vi "Shared Variable Main Page.vi"(8 "error in (no error)":errorcluster, 11 "Node Ptr":T1 format="%.0x") -> (0 "error out":errorcluster)   [LabVIEW 2012, in "Shared Variable Custom Device.lvlib"]
uses:
  Shared Variable Custom Device.lvlib
  <vilib>/NI Veristand/Custom Device API/Custom Device Item Ref.ctl
  <vilib>/NI Veristand/Custom Device API/Custom Device API.lvlib
panel:
  in  "Timeout (ms)":i32
  in  "IP Address":string
  in  "Header":cluster{"Section Name":string}={"Section Name"="Custom Device Item Settings"}
  in  "Description":string
  in  "Name":string
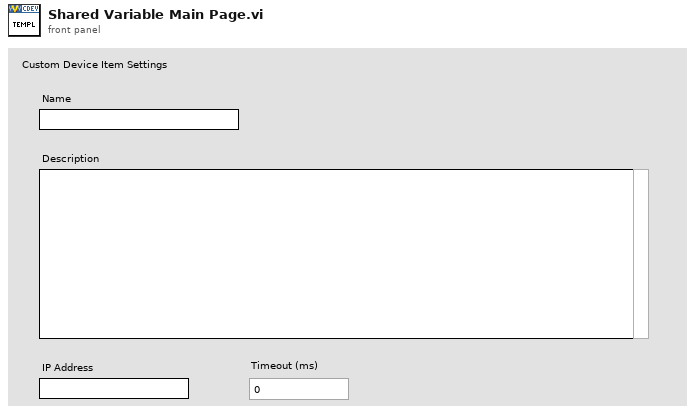
[diagram p1: front panel]
types:
  T1 = typedef "Custom Device API.lvlib/Custom Device Item Ref.ctl" = u64
  T2 = typedef "Custom Device API.lvlib/Custom Device Item Info.ctl" = cluster{"Name":string, "Is Channel":bool, "GUID":string, "Is Waveform":bool}
  T3 = typedef "Custom Device API.lvlib/Custom Device Commands.ctl" = enum16{"Default", "Item renamed", "Shutdown", "Dynamic button pressed"}
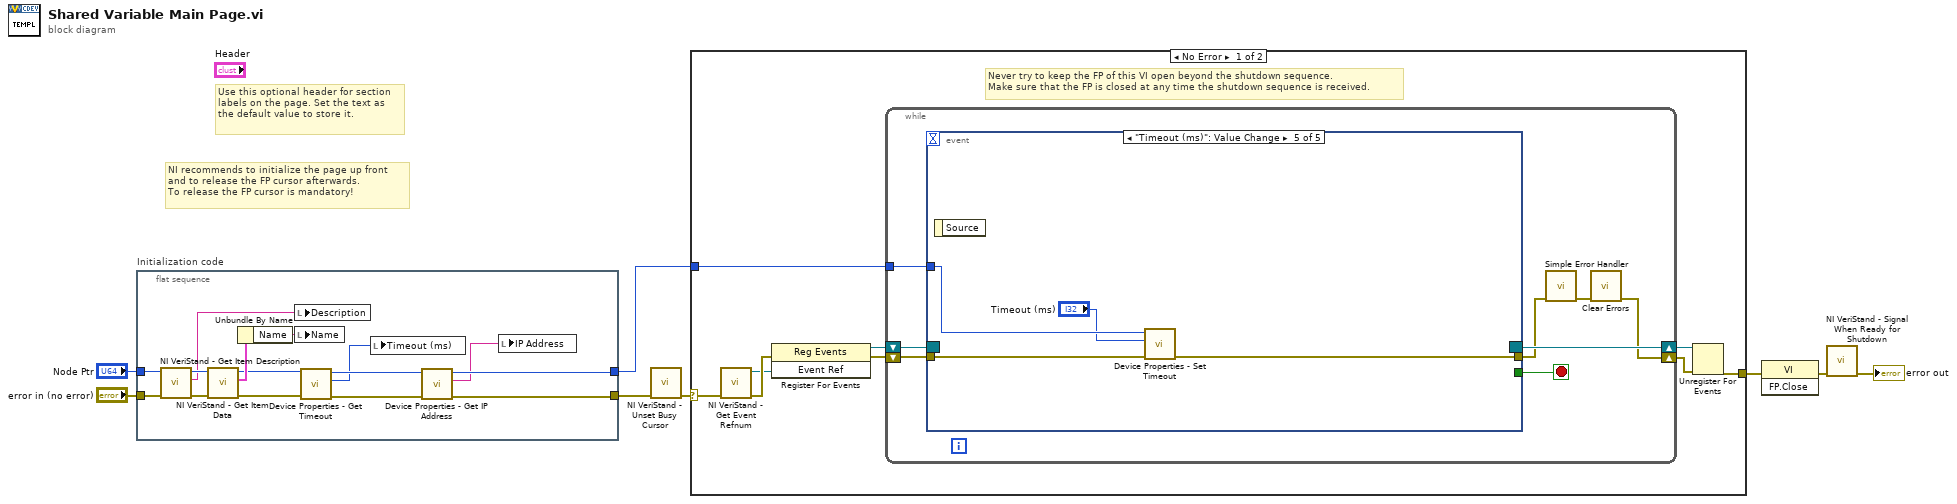
[diagram p0: block diagram]
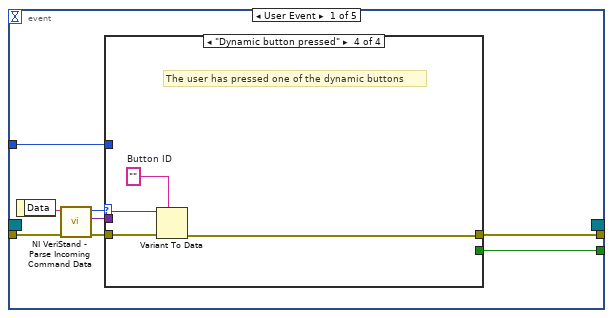
[diagram p2: hidden frame]
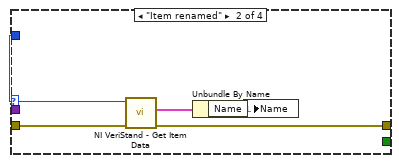
[diagram p4: hidden frame]
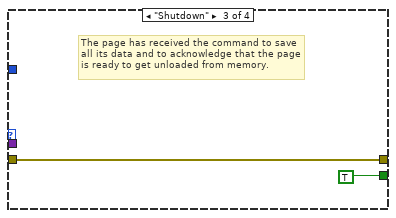
[diagram p5: hidden frame]
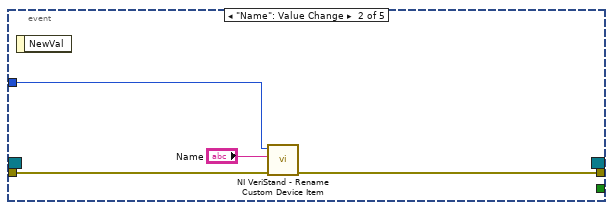
[diagram p6: hidden frame]
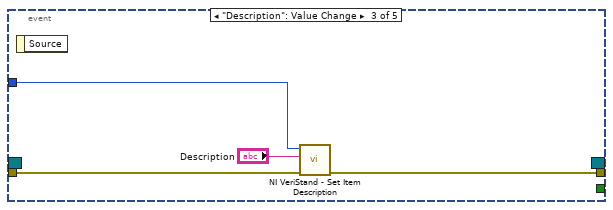
[diagram p7: hidden frame]
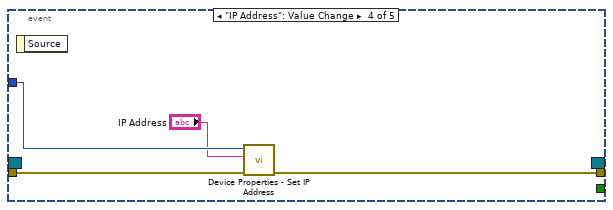
[diagram p8: hidden frame]
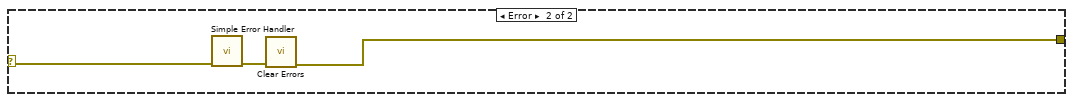
[diagram p9: hidden frame]
diagram:
  # "Use this optional header for section labels on the page. Set the text as the default value to store it."
  # "NI recommends to initialize the page up front\nand to release the FP cursor afterwards.\nTo release the FP cursor is mandatory!"
  n1 = flat-sequence "Initialization code" {
    tunnel: "error in (no error)" -> [w22]
    tunnel: "Node Ptr" -> [w21]
    tunnel: [w10] -> w4
    tunnel: [w11] -> w1
    frame #0 {
      n2 = call <vilib>:"NI VeriStand - Get Item Description.vi"("error in (no error)"=w22, "Item Ref in"=w21) -> ("error out"=w19:errorcluster, "Description"=w20:string, "Item Ref out"=w23:T1)  [unwired: 7 out]
      n3 = call <vilib>:"NI VeriStand - Get Item Data.vi"("error in (no error)"=w19, "Item Ref in"=w23) -> ("error out"=w15:errorcluster, "Item Info"=w18:T2, "Item Ref out"=w16:T1)  [unwired: 7 out]
      n4 = Unbundle By Name(w18) -> ("Name"=w17:string)
      n5 = local write "Description"(w20) -> ()
      n6 = local write "Name"(w17) -> ()
      n7 = call "Device Properties - Get Timeout.vi"("error in (no error)"=w15, "Device Ref in"=w16) -> ("error out"=w14:errorcluster, "IP Address"=w12:i32, "Device Ref out"=w13:T1)  [unwired: 7 in]
      n8 = local write "Timeout (ms)"(w12) -> ()
      n9 = call "Device Properties - Get IP Address.vi"("error in (no error)"=w14, "Device Ref in"=w13) -> ("error out"=w10:errorcluster, "IP Address"=w9:string, "Device Ref out"=w11:T1)  [unwired: 7 in]
      n10 = local write "IP Address"(w9) -> ()
    }
  }
  n11 = call <vilib>:"NI VeriStand - Unset Busy Cursor.vi"("error in (no error)"=w4) -> ("error out"=w3:errorcluster)  [unwired: 10 out]
  n12 = case shown="No Error" w3 {
    selector: w3 -> [w24 w79]
    tunnel: [w29 w77] -> w8
    tunnel: w1 -> [w25 _]
    frame No Error {
      # "Never try to keep the FP of this VI open beyond the shutdown sequence.\nMake sure that the FP is closed at any time the shutdown sequence is received."
      n13 = call <vilib>:"NI VeriStand - Get Event Refnum.vi"("error in (no error)"=w24) -> ("error out"=w32:errorcluster, "Event Ref"=w28:refnum<user-event>)  [unwired: 9 out]
      n14 = register-events(error in=w32, w28) -> (reference out=w26:refnum<event-registration>, error out=w27:errorcluster)  [unwired: 1 in]
      n15 = while {
        tunnel: w25 -> [w36]
        shift-right: [w33] -> w30
        shift-left: w27 -> [w39]
        shift-right: [w40] -> w31
        shift-left: w26 -> [w38]
        stop <- w37 stop-if-true
        n16 = event shown="[4] \"Timeout (ms)\": Value Change" {
          selector: w38 -> [_ _ _ _ _]
          dyn-events: [_ _ _ _ _] -> w40
          timeout: _ -> [_ _ _ _ _]
          tunnel: w39 -> [w48 w64 w67 w72 w76]
          tunnel: [w44 _ _ _ _] -> w37
          tunnel: [w43 w63 w66 w69 w73] -> w35
          tunnel: w36 -> [w42 w62 w68 w71 w75]
          event User Event {
            n17 = event-data() -> ("Data"=w47:string)  [unwired: 1 out]
            n18 = call <vilib>:"NI VeriStand - Parse Incoming Command Data.vi"("error in (no error)"=w48, "Incoming data"=w47) -> ("error out"=w46:errorcluster, "Outgoing data"=w41:variant, "Action"=w45:T3)  [unwired: 7 out]
            n19 = case shown="\"Dynamic button pressed\"" w45 {
              tunnel: w46 -> [w49 w54 w55 w60]
              tunnel: [_ _ TRUE _] -> w44
              tunnel: [w49 w51 w55 w57] -> w43
              tunnel: w42 -> [_ w53 _ _]
              tunnel: w41 -> [_ _ _ w59]
              frame "Default", Default {
              }
              frame "Item renamed" {
                n20 = call <vilib>:"NI VeriStand - Get Item Data.vi"("error in (no error)"=w54, "Item Ref in"=w53) -> ("error out"=w51:errorcluster, "Item Info"=w52:T2)  [unwired: 8 out]
                n21 = Unbundle By Name(w52) -> ("Name"=w50:string)
                n22 = local write "Name"(w50) -> ()
              }
              frame "Shutdown" {
                # "The page has received the command to save all its data and to acknowledge that the page is ready to get unloaded from memory."
              }
              frame "Dynamic button pressed" {
                w58 = ""  # Button ID
                # "The user has pressed one of the dynamic buttons"
                n23 = Variant To Data(error in=w60, type=w58, Variant=w59) -> (error out=w57:errorcluster)  [unwired: 1 out]
              }
            }
          }
          event "Name": Value Change {
            n24 = event-data() -> ()  [unwired: 2 out]
            n25 = call <vilib>:"NI VeriStand - Rename Custom Device Item.vi"("error in (no error)"=w64, "New Name"="Name", "Item Ref in"=w62) -> ("error out"=w63:errorcluster)  [unwired: 1 in, 7 out]
          }
          event "Description": Value Change {
            n26 = event-data() -> ()  [unwired: 2 out]
            n27 = call <vilib>:"NI VeriStand - Set Item Description.vi"("error in (no error)"=w67, "Description"="Description", "Item Ref in"=w68) -> ("error out"=w66:errorcluster)  [unwired: 8 out]
          }
          event "IP Address": Value Change {
            n28 = event-data() -> ()  [unwired: 2 out]
            n29 = call "Device Properties - Set IP Address.vi"("error in (no error)"=w72, "IP Address"="IP Address", "Device Ref in"=w71) -> ("error out"=w69:errorcluster)  [unwired: 7 in, 1 out]
          }
          event "Timeout (ms)": Value Change {
            n30 = event-data() -> ()  [unwired: 2 out]
            n31 = call "Device Properties - Set Timeout.vi"("error in (no error)"=w76, "IP Address"="Timeout (ms)", "Device Ref in"=w75) -> ("error out"=w73:errorcluster)  [unwired: 7 in, 1 out]
          }
        }
        n32 = call <vilib>:"Simple Error Handler.vi"("error in (no error)"=w35) -> ("error out"=w34:errorcluster)  [unwired: 1 in, 7 out]
        n33 = call <vilib>:"Clear Errors.vi"("error in (no error)"=w34) -> ("error out"=w33:errorcluster)  [unwired: 6 out]
      }
      n34 = Unregister For Events(event registration refnum=w31, error in=w30) -> (error out=w29:errorcluster)
    }
    frame Error {
      n35 = call <vilib>:"Simple Error Handler.vi"("error in (no error)"=w79) -> ("error out"=w78:errorcluster)  [unwired: 1 in, 7 out]
      n36 = call <vilib>:"Clear Errors.vi"("error in (no error)"=w78) -> ("error out"=w77:errorcluster)  [unwired: 6 out]
    }
  }
  n37 = invoke class="VI" method="FP.Close"(error in=w8) -> (error out=w7:errorcluster)  [unwired: 2 in, 2 out]
  n38 = call <vilib>:"NI VeriStand - Signal When Ready for Shutdown.vi"("error in (no error)"=w7) -> ("error out"=→"error out":errorcluster)  [unwired: 10 out]
